vi "Run.vi"(8 "error in (no error)":errorcluster, 11 "MCCW ACLR in":refnum<class "MCCW ACLR.lvclass">) -> (0 "error out":errorcluster, 1 "Parameters":cluster{"Name":string, "Value":string}[](array[cluster]), 2 "Cancled":bool, 3 "MCCW ACLR out":refnum<class "MCCW ACLR.lvclass">)   [LabVIEW 2020, in "MCCW ACLR.lvclass"]
doc: "This is the main test vi. It is here that the test is implemented."
uses:
  MCCW ACLR.lvclass
  C:/Sandbox/RF Bench/Source Code/WiSpry Test Framework/Measurements/Measurement.lvclass
  Controls/Run States.ctl
  MCCW ACLR.lvclass/MCCW ACLR.ctl
  Instruments/Spectrum Analyzer/Spectrum Analyzer.lvclass/Spectrum Analyzer.ctl
  Measurement.lvclass/Measurement.ctl
  Devices/Controls/Change setting mode enum.ctl
  Support VI/Update parameters (single).vi
  Devices/Device.lvclass
  Instruments/Spectrum Analyzer/Spectrum Analyzer.lvclass
  Instruments/Vector Signal Generator/Vector Signal Generator.lvclass
  Measurement.lvclass
  XML Handler/XML Handler.lvclass
  Devices/PIC-device/PIC-Device.lvclass
panel:
  out "Number of Carriers":i32
  out "Device Parameters":string
  in  "Cancel Button":bool
  out "Current Frequency [Hz]":dbl format="%#_6p"
  out "Current Power [dBm]":dbl
  out "Estimated finish time":timestamp format="%<%X>T"
  out "XY Graph":cluster{dbl[], dbl[]}[](graph)
  out "Progress":u8(slide) scale=0.0..100.0
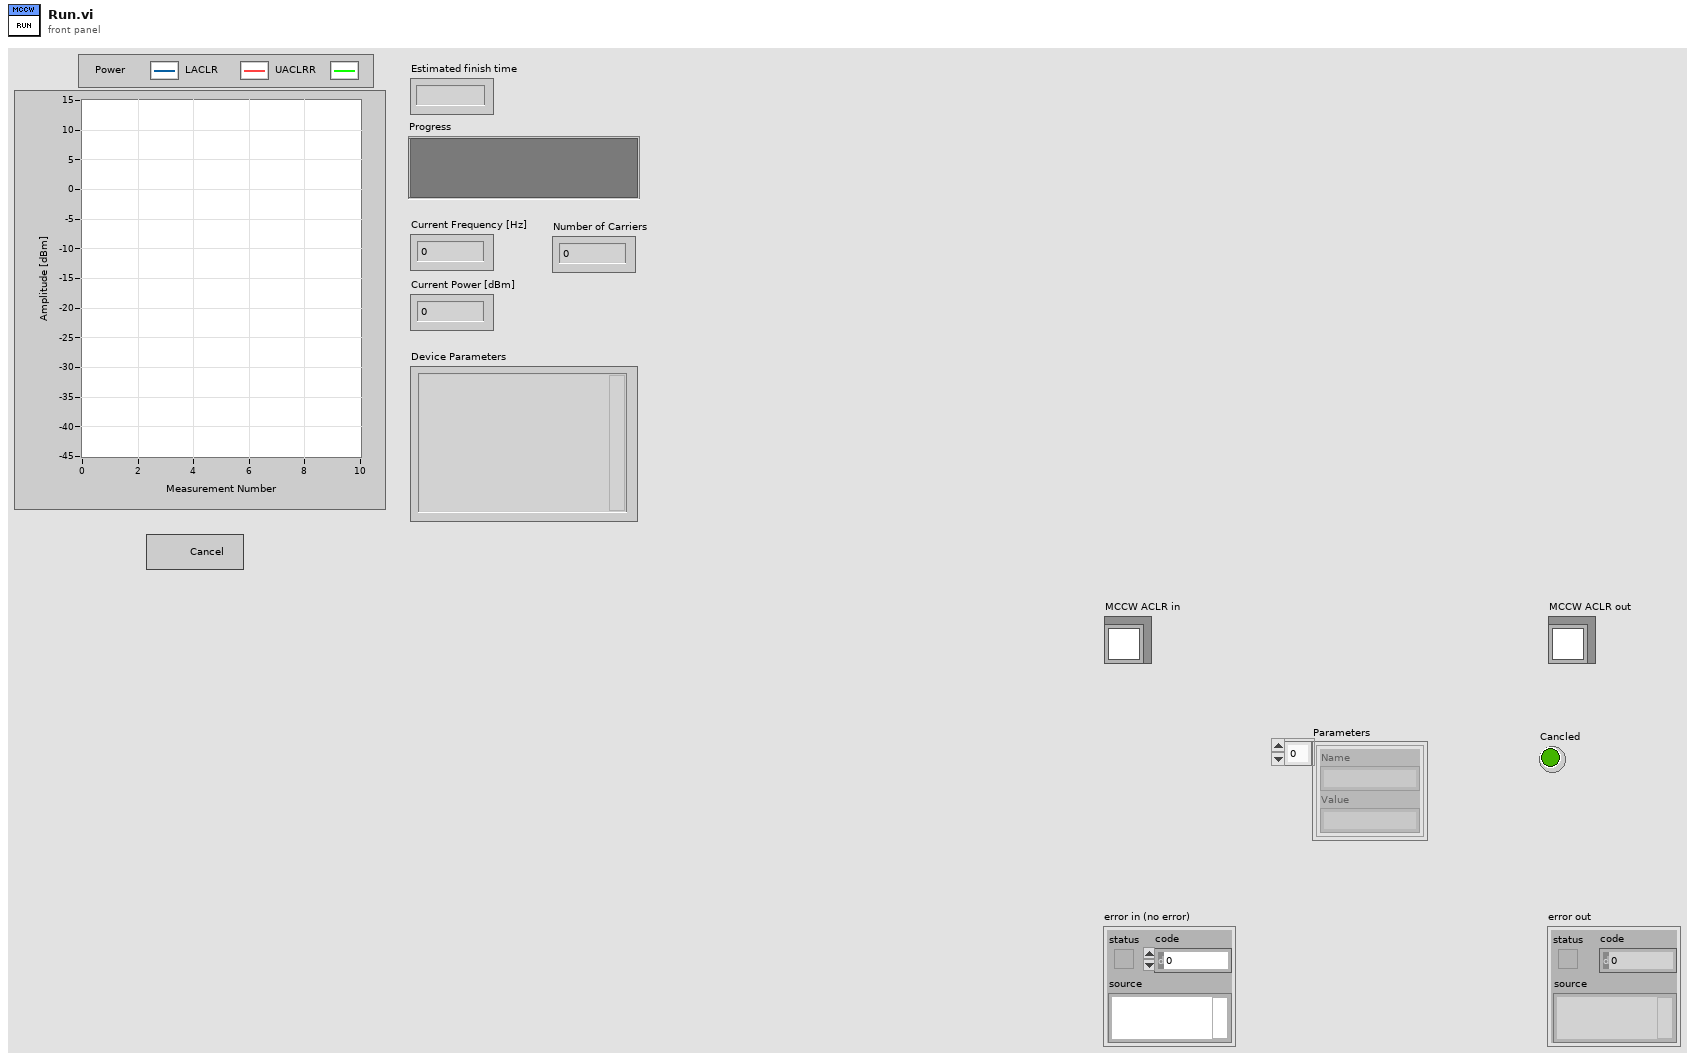
[diagram p1: front panel]
types:
  T1 = typedef "MCCW ACLR.lvclass/Run States.ctl" = enum16{"Init", "Set Frequency", "Set Power", "Set Carriers", "Set Device", "Set Measurement Number", "Measure", "Done"}
  T2 = typedef "PIC-Device.lvclass/Change setting mode enum.ctl" = enum16{"Init", "Next", "Reset"}
  T3 = typedef "MCCW ACLR.lvclass/ACLR configuration.ctl" = cluster{"Frequency":cluster{"Cluster ":cluster{"From":dbl, "To":dbl, "Step":dbl}, "Array":dbl[], "Use Array":bool}, "Power":cluster{"Cluster ":cluster{"From":dbl, "To":dbl, "Step":dbl}, "Array":dbl[], "Use Array":bool}, "Carriers":cluster{"Cluster ":cluster{"From":dbl, "To":dbl, "Step":dbl}, "Array":dbl[], "Use Array":bool}, "Phase Value":dbl, "Number of Measurements":u32, "Use random phase":bool, "Signal BW [MHz] ":dbl}
  T4 = cluster{"List":dbl[], "Index":i32, "Last":bool, "BW [MHz]":dbl}
  T5 = cluster{"Number of Measurements":u32, "Current Measurement":u32, "Last":bool}
  T6 = typedef "XML Handler.lvclass/Result Cluster.ctl" = cluster{"Name":string, "Value":string}
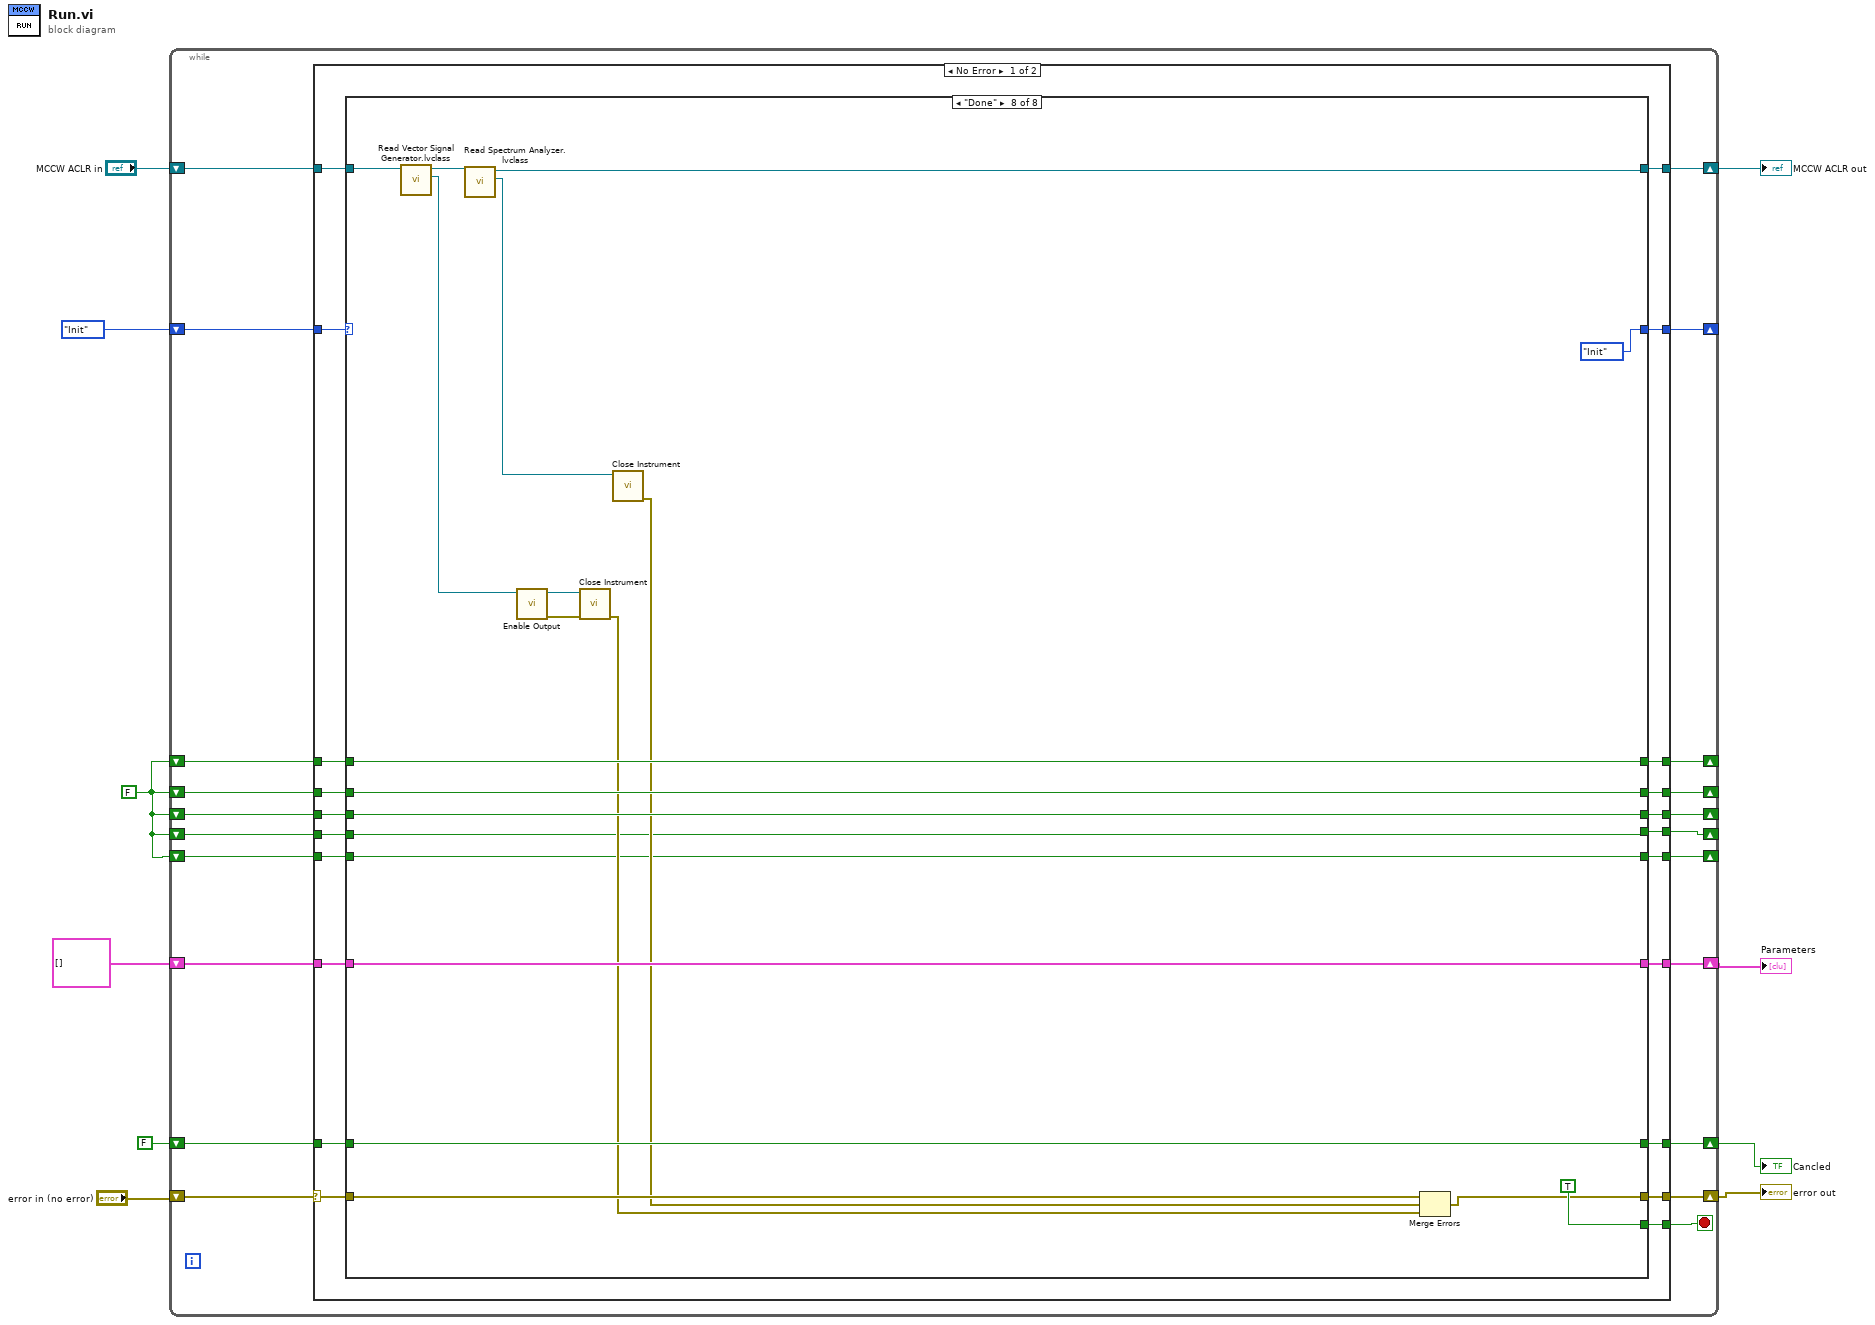
[diagram p0: block diagram]
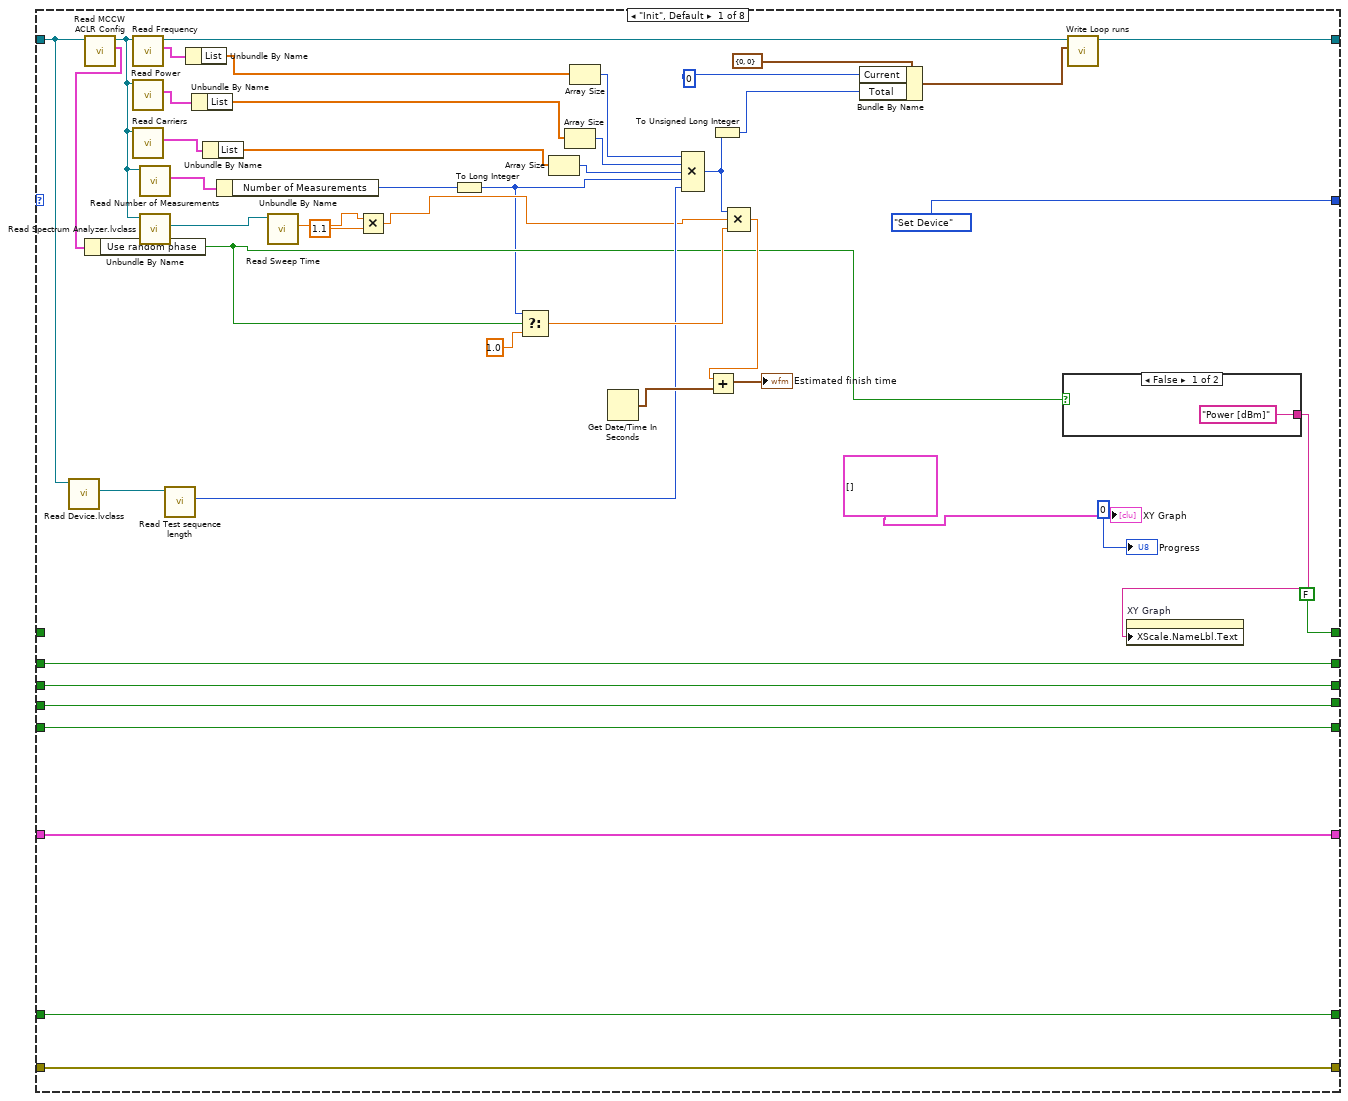
[diagram p2: hidden frame]
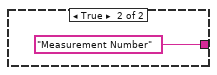
[diagram p3: hidden frame]
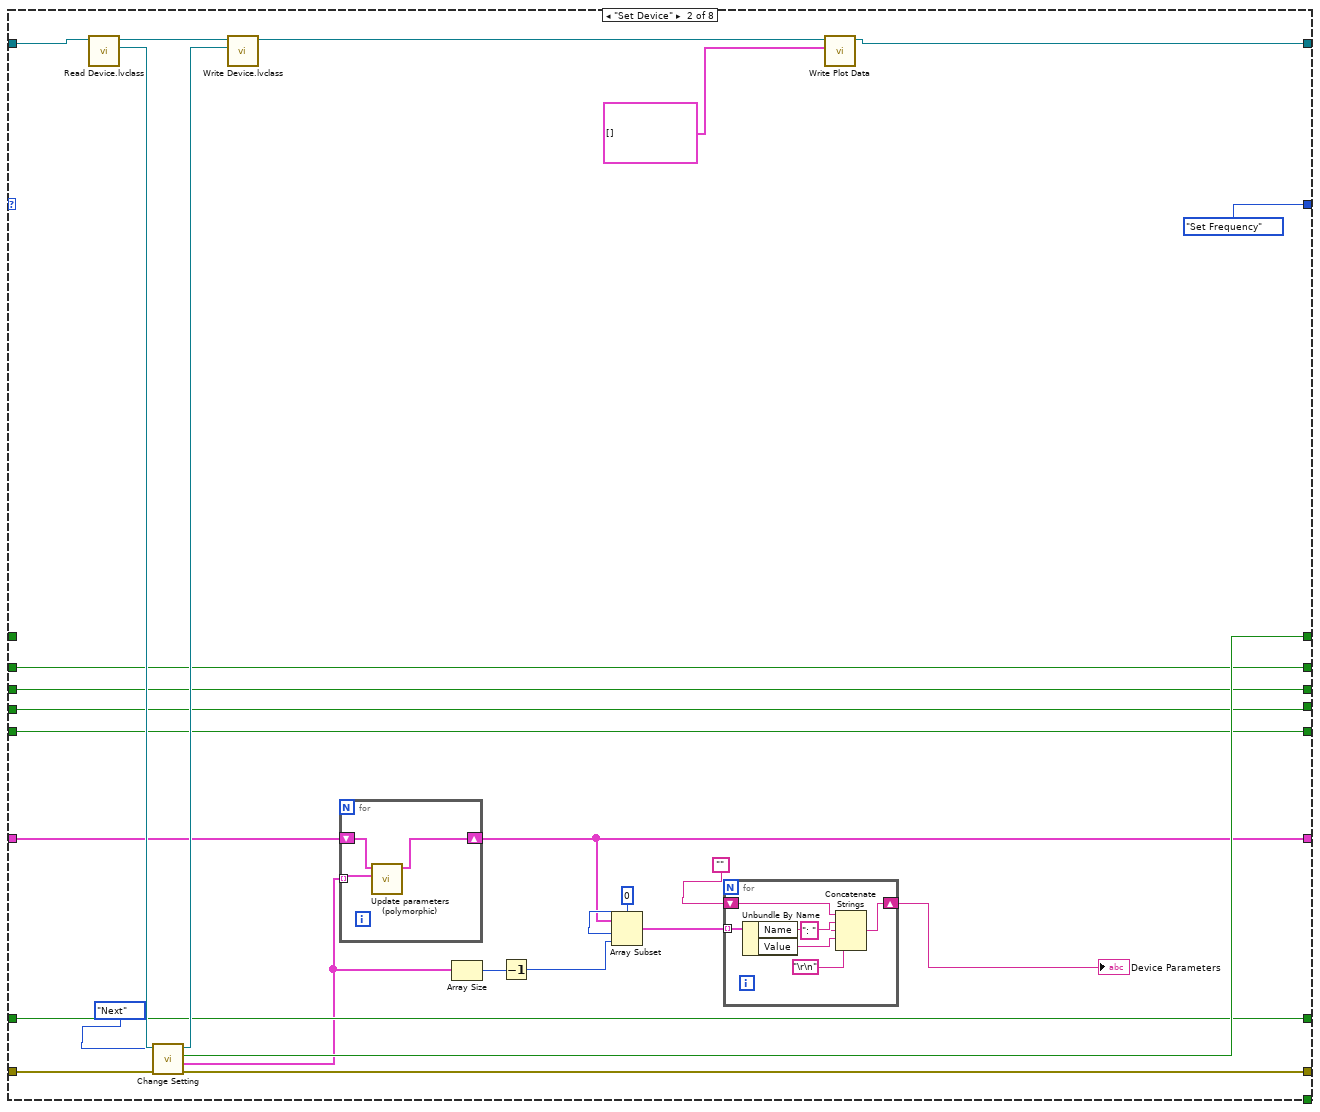
[diagram p4: hidden frame]
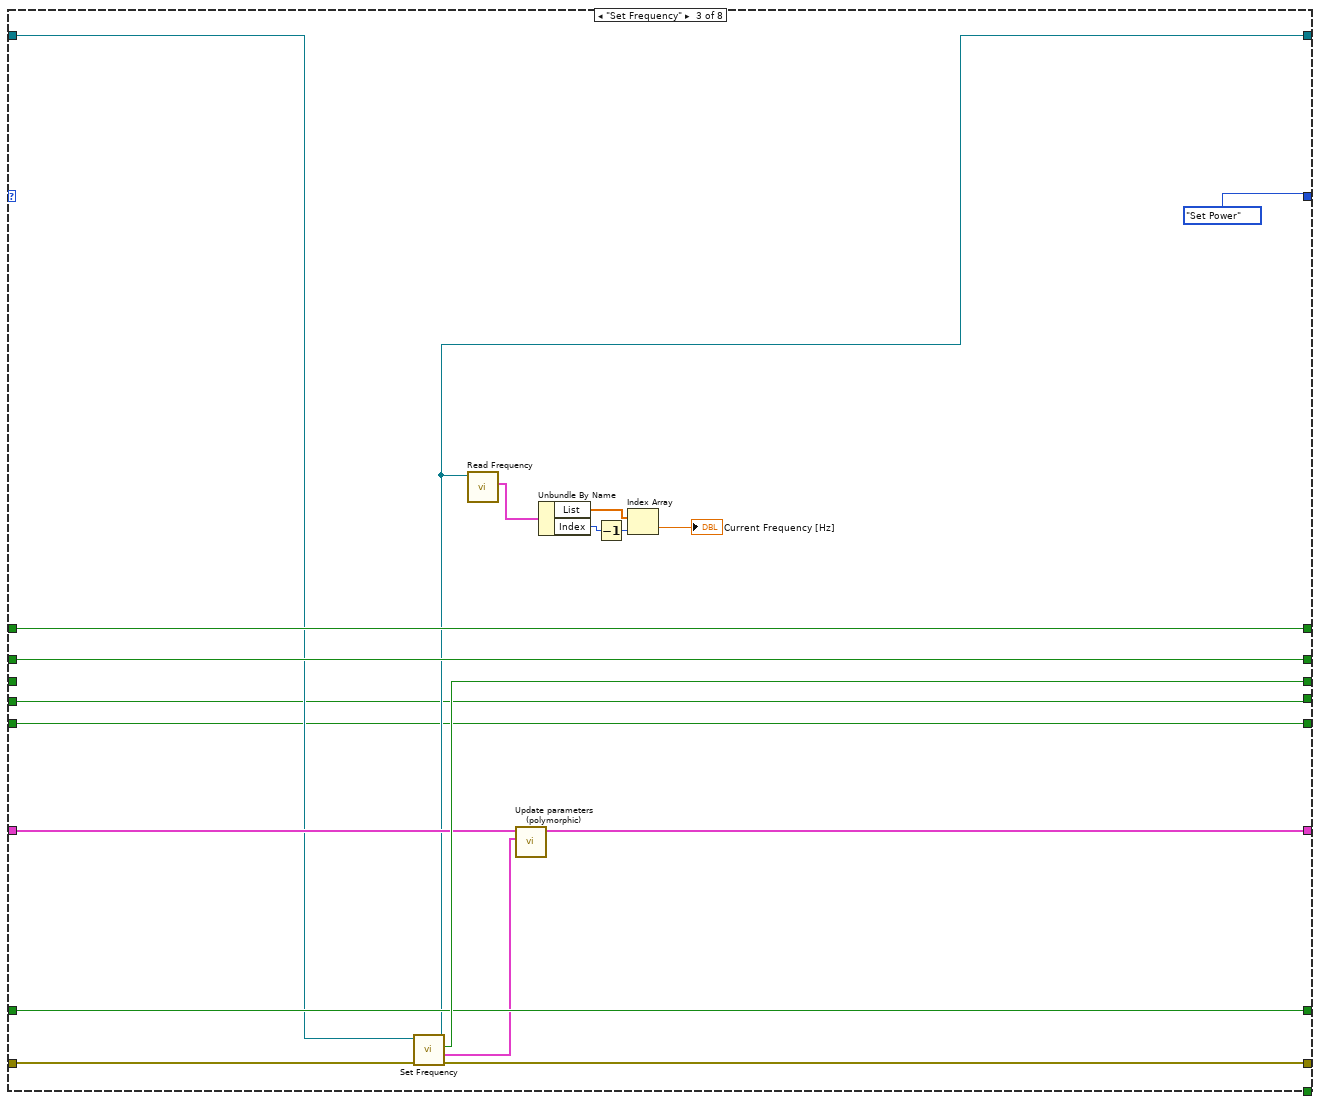
[diagram p5: hidden frame]
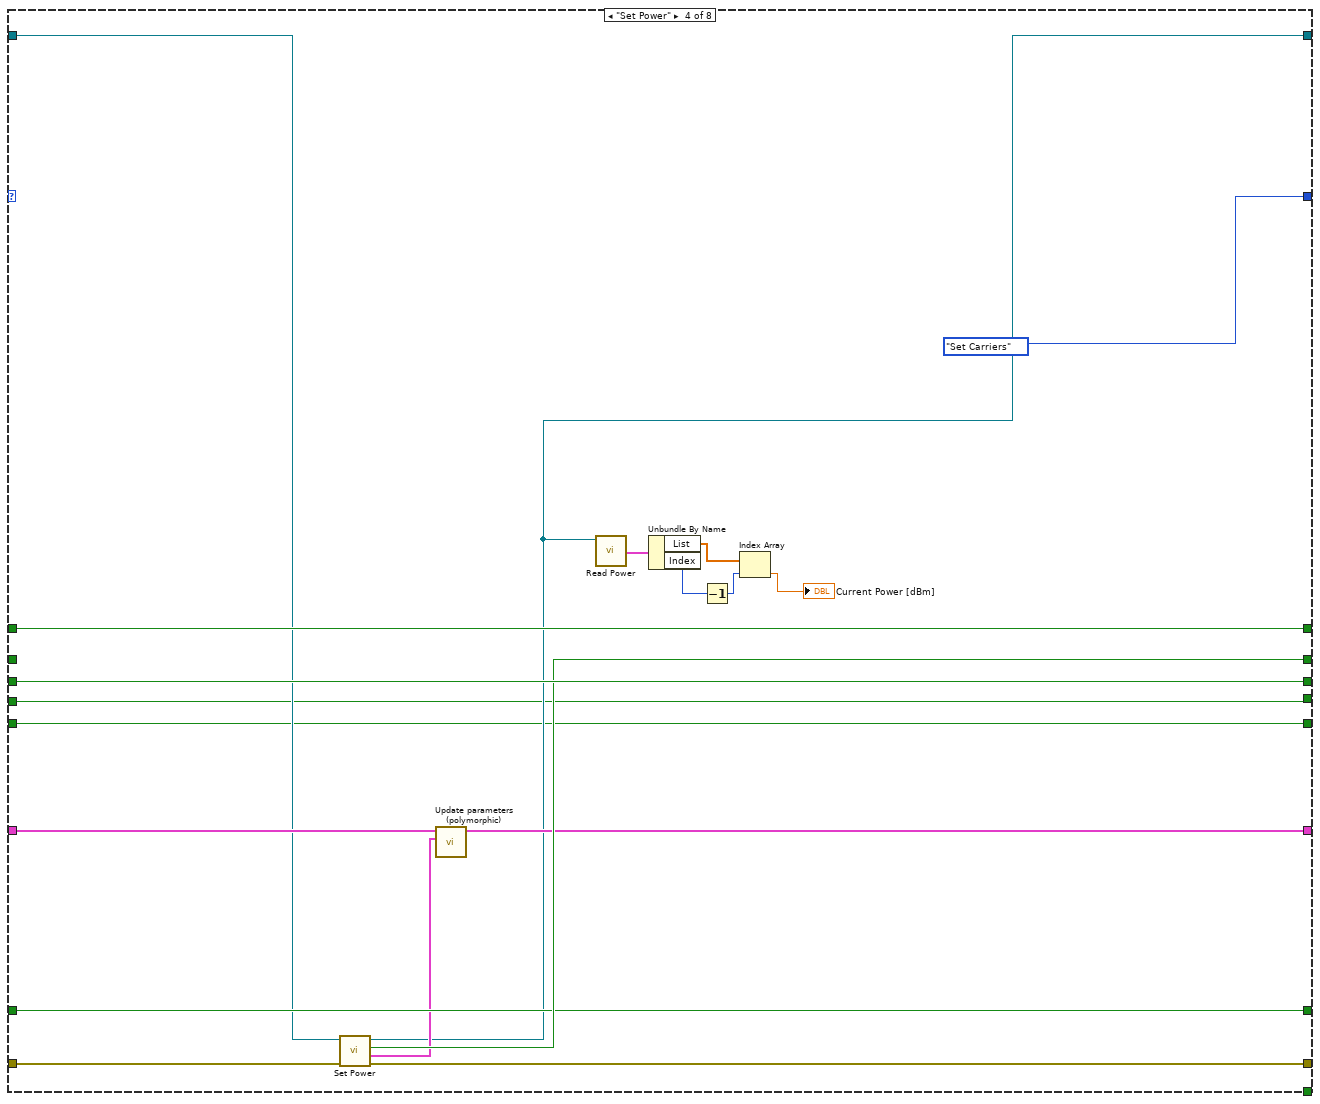
[diagram p6: hidden frame]
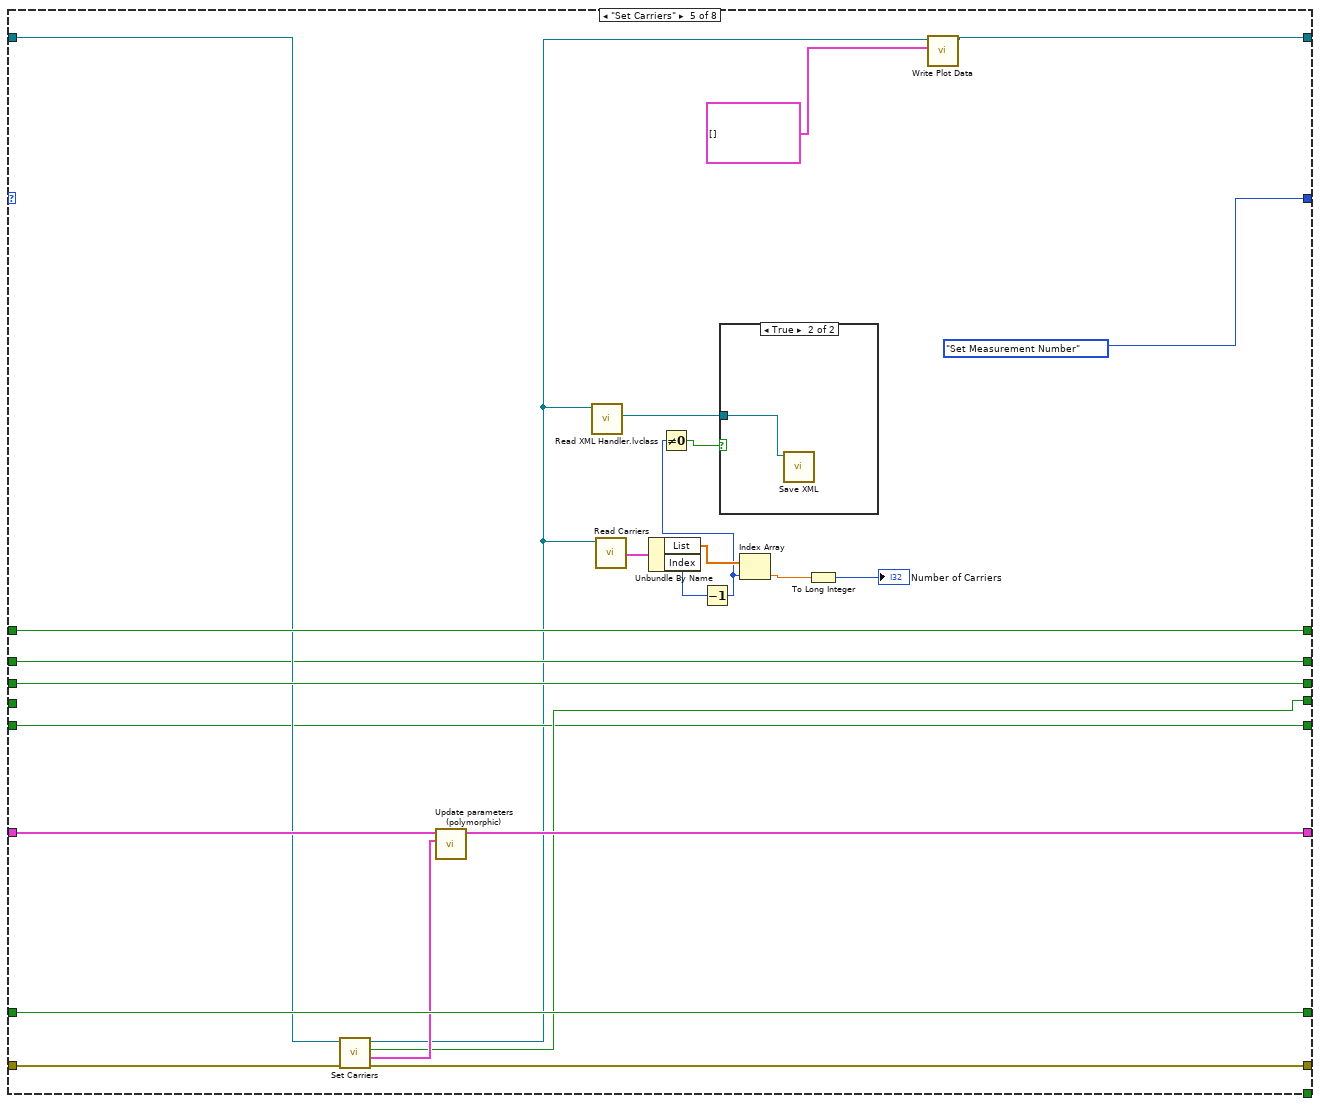
[diagram p7: hidden frame]
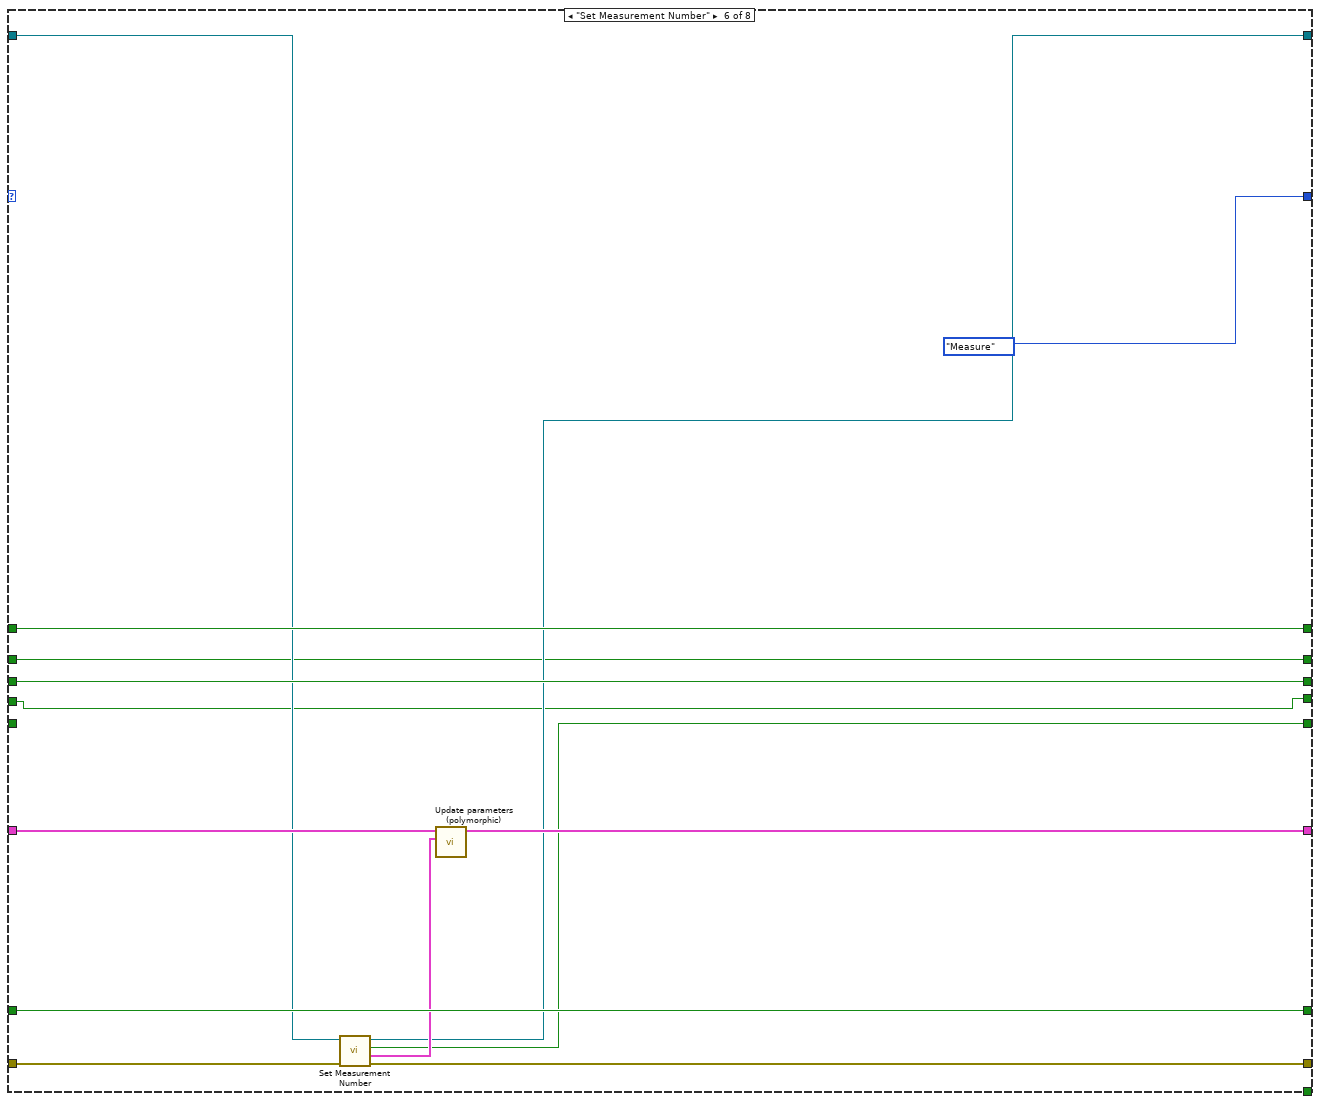
[diagram p9: hidden frame]
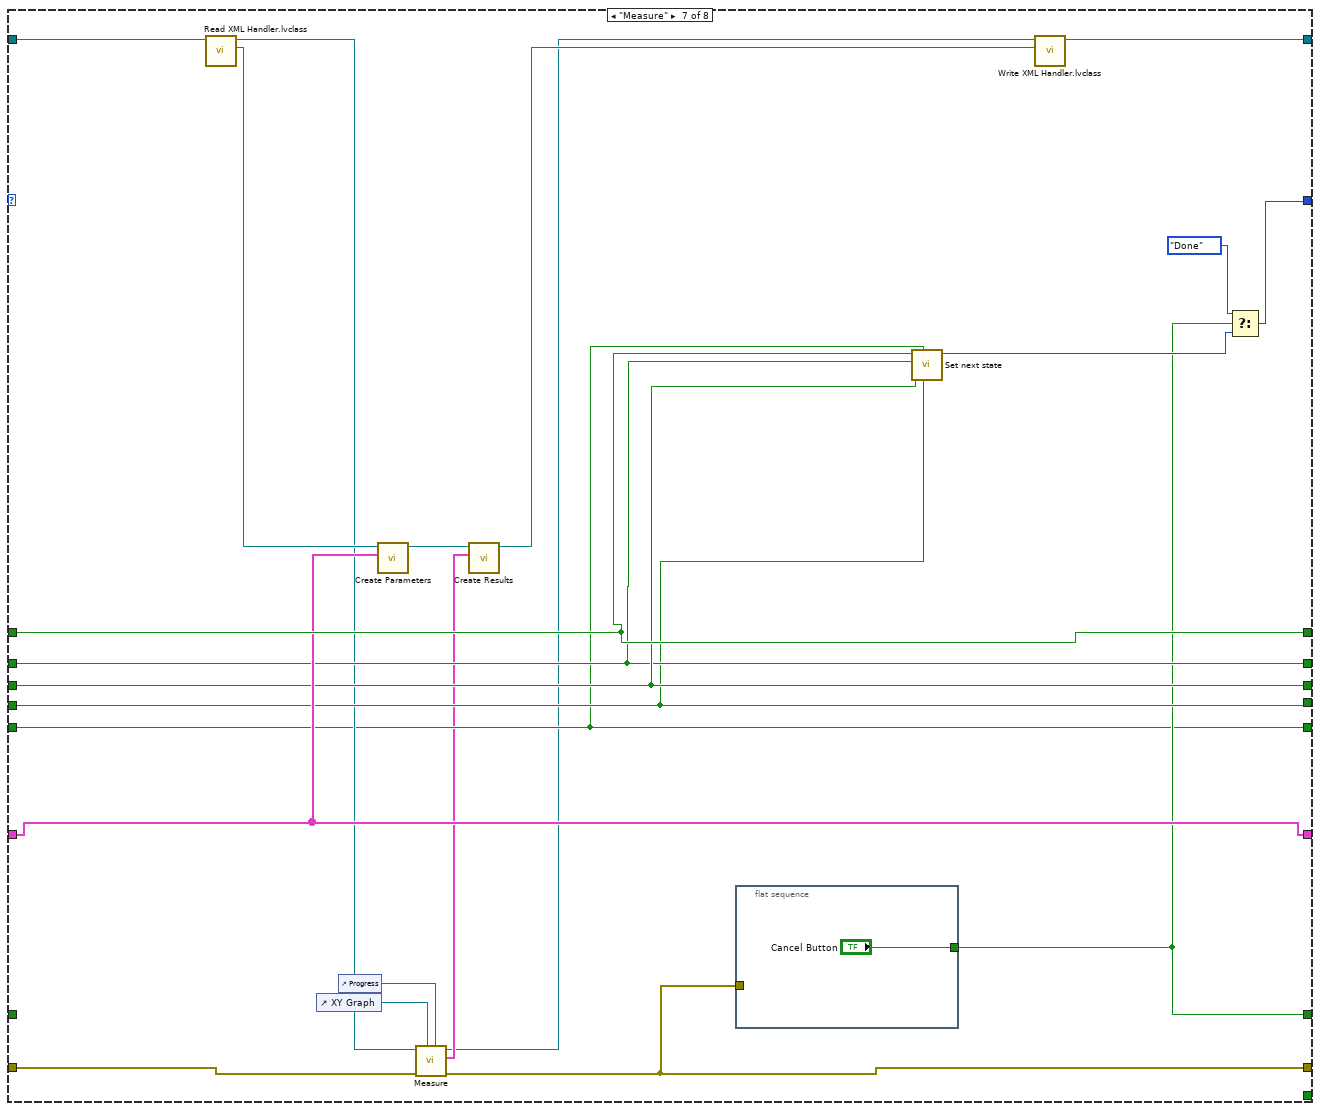
[diagram p10: hidden frame]
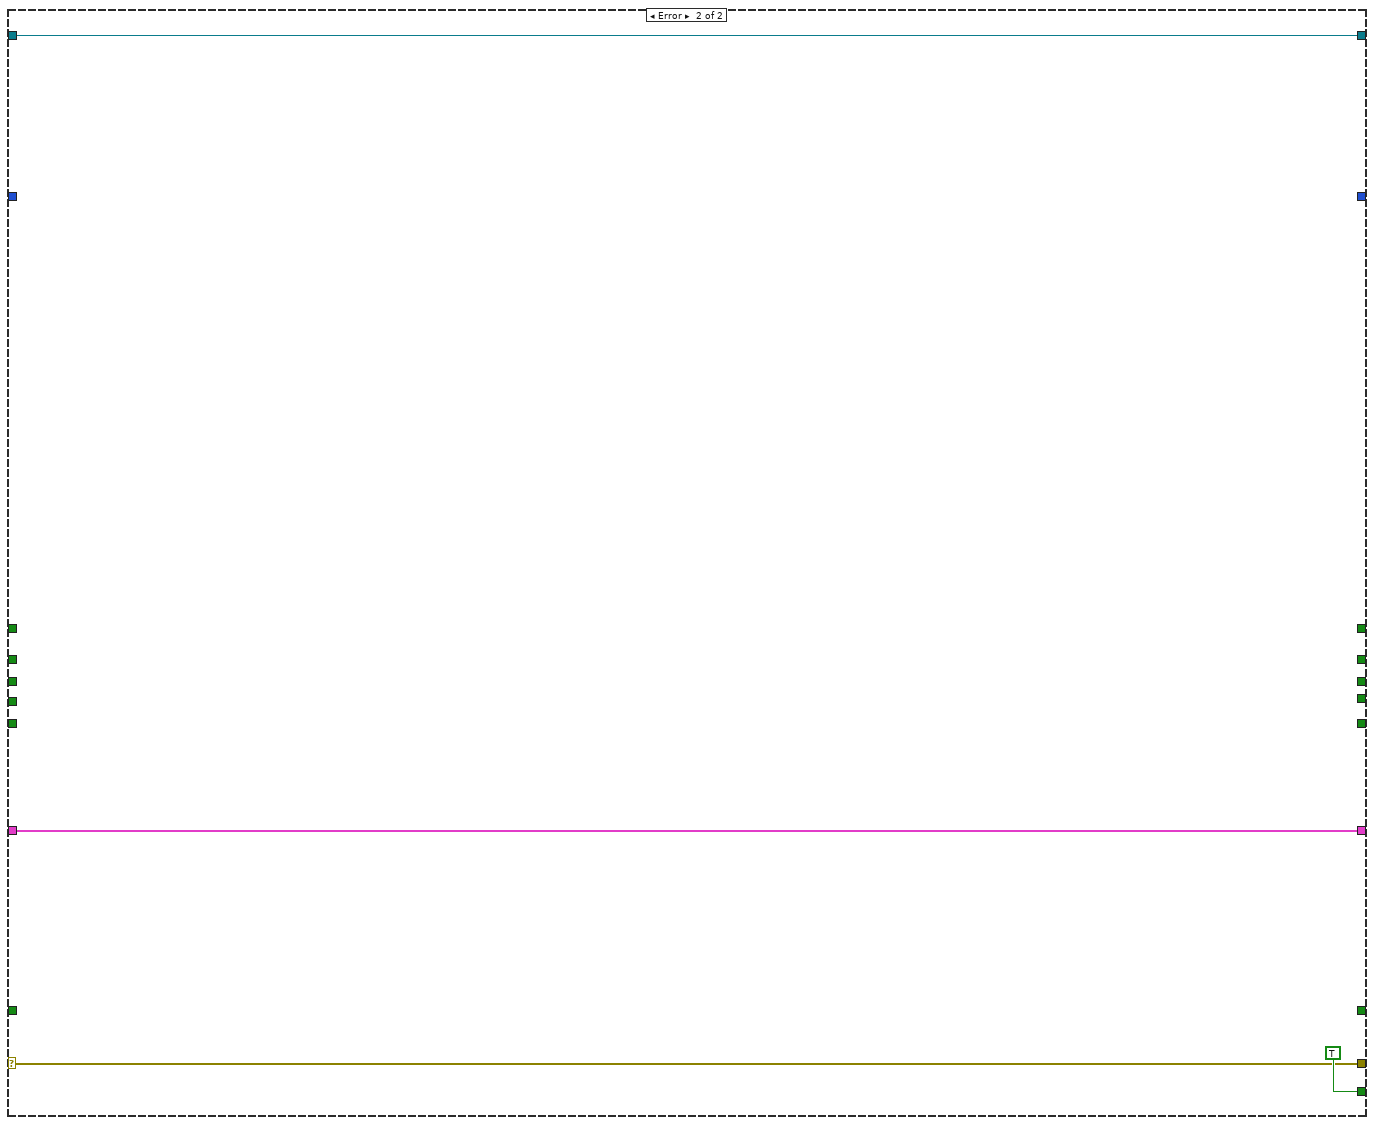
[diagram p11: hidden frame]
diagram:
  w5 = FALSE
  n1 = while {
    shift-right: [w28] -> w4
    shift-left: "error in (no error)" -> [w31]
    shift-right: [w14] -> _
    shift-left: Run_States."Init" ("Run States") -> [w30]
    shift-right: [w27] -> _
    shift-left: w5 -> [w26]
    shift-right: [w23] -> _
    shift-left: w5 -> [w25]
    shift-right: [w22] -> _
    shift-left: w5 -> [w24]
    shift-right: [w21] -> w3
    shift-left: FALSE ("Cancel Button") -> [w20]
    shift-right: [w18] -> w1
    shift-left: cluster{"Name":string, "Value":string}[] [] ("Parameters") -> [w19]
    shift-right: [w13] -> w7
    shift-left: "MCCW ACLR in" -> [w17]
    shift-right: [w15] -> _
    shift-left: w5 -> [w16]
    shift-right: [w11] -> _
    shift-left: w5 -> [w12]
    stop <- w29 stop-if-true
    n2 = case shown="No Error" w31 {
      selector: w31 -> [w50 w259]
      tunnel: w17 -> [w52 w257]
      tunnel: w30 -> [w51 _]
      tunnel: [w32 w257] -> w13
      tunnel: [w49 TRUE] -> w29
      tunnel: [w48 w259] -> w28
      tunnel: [w47 _] -> w27
      tunnel: w26 -> [w46 _]
      tunnel: [w45 _] -> w14
      tunnel: w25 -> [w44 _]
      tunnel: w24 -> [w43 _]
      tunnel: [w42 _] -> w23
      tunnel: [w41 _] -> w22
      tunnel: [w40 _] -> w21
      tunnel: w20 -> [w39 _]
      tunnel: w19 -> [w38 w258]
      tunnel: [w37 w258] -> w18
      tunnel: w16 -> [w36 _]
      tunnel: [w35 _] -> w15
      tunnel: w12 -> [w34 _]
      tunnel: [w33 _] -> w11
      frame No Error {
        n3 = case shown="\"Done\"" w51 {
          tunnel: w52 -> [w62 w126 w139 w160 w186 w205 w235 w241]
          tunnel: [w77 w103 w141 w159 w179 w204 w233 w238] -> w32
          tunnel: w50 -> [w79 w123 w153 w172 w196 w211 w222 w248]
          tunnel: [_ _ _ _ _ _ _ TRUE] -> w49
          tunnel: [w79 w116 w150 w169 w194 w209 w214 w245] -> w48
          tunnel: [FALSE ("Last setting") w121 w155 w174 w198 w213 w232 w256] -> w47
          tunnel: w46 -> [_ _ w155 w174 w198 w213 w232 w256]
          tunnel: [Run_States."Set Device" ("Run States") Run_States."Set Frequency" ("Run States") Run_States."Set Power" ("Run States") Run_States."Set Carriers" ("Run States") Run_States."Set Measurement Number" ("Run States") Run_States."Measure" ("Run States") w230 Run_States."Init" ("Run States")] -> w45
          tunnel: w44 -> [w91 w120 w154 _ w183 w202 w225 w255]
          tunnel: w43 -> [w90 w119 _ w173 w197 w212 w226 w254]
          tunnel: [w91 w120 w154 w171 w183 w202 w225 w255] -> w42
          tunnel: [w90 w119 w152 w173 w197 w212 w226 w254] -> w41
          tunnel: [w87 w118 w151 w170 w195 w210 w220 w252] -> w40
          tunnel: w39 -> [w87 w118 w151 w170 w195 w210 _ w252]
          tunnel: w38 -> [w82 w115 w149 w168 w193 w208 w227 w251]
          tunnel: [w82 w111 w148 w167 w192 w207 w227 w251] -> w37
          tunnel: w36 -> [w64 w102 w138 w157 _ w201 w224 w244]
          tunnel: [w64 w102 w138 w157 w184 w201 w224 w244] -> w35
          tunnel: w34 -> [w61 w101 w137 w156 w181 _ w217 w242]
          tunnel: [w61 w101 w137 w156 w181 w200 w217 w242] -> w33
          frame "Init", Default {
            n4 = call "Read Device.lvclass.vi"("Measurements in"=w62) -> ("Device.lvclass"=w92:refnum<class "Device.lvclass">)  [unwired: 9 in, 1 out]
            n5 = call "Read MCCW ACLR Config.vi"("MCCW ACLR in"=w62) -> ("MCCW ACLR Config"=w75:T3, "MCCW ACLR out"=w57:refnum<class "MCCW ACLR.lvclass">)  [unwired: 9 in]
            n6 = Unbundle By Name(w75) -> ("Use random phase"=w76:bool)
            n7 = call "Read Frequency.vi"("MCCW ACLR in"=w57) -> ("Frequency"=w74:cluster{"List":dbl[], "Index":i32, "Last":bool}, "MCCW ACLR out"=w63:refnum<class "MCCW ACLR.lvclass">)  [unwired: 9 in]
            n8 = call "Read Power.vi"("MCCW ACLR in"=w57) -> ("Power"=w73:cluster{"List":dbl[], "Index":i32, "Last":bool})  [unwired: 9 in, 1 out]
            n9 = call "Read Carriers.vi"("MCCW ACLR in"=w57) -> ("Carriers"=w72:T4)  [unwired: 9 in, 1 out]
            n10 = call "Read Number of Measurements.vi"("MCCW ACLR in"=w57) -> ("Number of Measurements"=w56:T5)  [unwired: 9 in, 1 out]
            n11 = call "Read Spectrum Analyzer.lvclass.vi"("MCCW ACLR in"=w57) -> ("Spectrum Analyzer.lvclass"=w67:refnum<class "Spectrum Analyzer.lvclass">)  [unwired: 9 in, 1 out]
            n12 = call-dynamic "Read Test sequence length.vi"("Device in"=w92) -> ("Test sequence length"=w93:i32)  [unwired: 8 in, 2 out]
            n13 = Unbundle By Name(w74) -> ("List"=w89:dbl[])
            n14 = Unbundle By Name(w73) -> ("List"=w88:dbl[])
            n15 = Unbundle By Name(w72) -> ("List"=w68:dbl[])
            n16 = Unbundle By Name(w56) -> ("Number of Measurements"=w55:u32)
            n17 = call "Read Sweep Time.vi"("Spectrum Analyzer in"=w67) -> ("Sweep Time"=w60:dbl)  [unwired: 9 in, 1 out]
            n18 = Multiply(x=w60, y=1.1) -> (x*y=w59:dbl)
            n19 = To Long Integer(number=w55) -> (32bit integer=w53:i32)
            n20 = Select(t=w53, s=w76, f=1.0) -> (s? t:f=w95:dbl)
            n21 = Array Size(array=w68) -> (size(s)=w69:i32)
            n22 = Array Size(array=w88) -> (size(s)=w70:i32)
            n23 = Array Size(array=w89) -> (size(s)=w71:i32)
            n24 = Get Date/Time In Seconds() -> (seconds since 1Jan1904=w98:timestamp)
            n25 = Compound Arithmetic op=MULTIPLY(w71, w70, w69, w53, w93) -> (w83:i32)
            n26 = To Unsigned Long Integer(number=w83) -> (unsigned 32bit integer=w54:u32)
            n27 = Compound Arithmetic op=MULTIPLY(w83, w59, w95) -> (w94:dbl)
            n28 = Add(x=w94, y=w98) -> (x+y=→"Estimated finish time":timestamp)
            n29 = Bundle By Name(cluster=cluster{"Current":u32, "Total":u32} {"Current"=0, "Total"=0} ("Loop runs"), "Current"=u32 0, "Total"=w54) -> (w84:cluster{"Current":u32, "Total":u32})
            n30 = case shown="False" w76 {
              tunnel: ["Power [dBm]" "Measurement Number"] -> w80
              frame False {
              }
              frame True {
              }
            }
            n31 = call "Write Loop runs.vi"("Loop runs"=w84, "Measurements in"=w63) -> ("Measurements out"=w77:refnum<class "MCCW ACLR.lvclass">)  [unwired: 9 in]
            n32 = property on="XY Graph" class="XYGraph (strict)"("XScale.NameLbl.Text"=w80) -> ()  [unwired: 2 in, 2 out]
            "XY Graph" <- cluster{dbl[], dbl[]}[] [] ("XY Graph")
            "Progress" <- u8 0 ("Progress")
          }
          frame "Set Device" {
            n33 = call "Read Device.lvclass.vi"("Measurements in"=w126) -> ("Device.lvclass"=w125:refnum<class "Device.lvclass">, "Measurements out"=w117:refnum<class "MCCW ACLR.lvclass">)  [unwired: 9 in]
            n34 = call-dynamic "Change Setting.vi"("error in (no error)"=w123, "Change setting mode"=Change_setting_mode_enum."Next", "Device in"=w125) -> ("error out"=w116:errorcluster, "Changes"=w114:cluster{"Name":string, "Value":string}[], "Last setting"=w121:bool, "Device out"=w122:refnum<class "Device.lvclass">)  [unwired: 5 in]
            n35 = call "Write Device.lvclass.vi"("Device.lvclass"=w122, "Measurements in"=w117) -> ("Measurements out"=w105:refnum<class "MCCW ACLR.lvclass">)  [unwired: 9 in]
            n36 = for {
              shift-right: [w135] -> w111
              shift-left: w115 -> [w136]
              tunnel: w114 -> [w134] mode=indexing
              n37 = call-poly "Update parameters (polymorphic).vi"("New Parameter"=w134, "Parameters"=w136) -> ("Parameters Out"=w135:cluster{"Name":string, "Value":string}[])  [unwired: 9 in]
            }
            n38 = Array Size(array=w114) -> (size(s)=w112:i32)
            n39 = Decrement(x=w112) -> (x-1=w107:i32)
            n40 = Array Subset(array=w111, index=0, length=w107) -> (w110:cluster{"Name":string, "Value":string}[])
            n41 = for {
              tunnel: w110 -> [w133] mode=indexing
              shift-right: [w127] -> w108
              shift-left: "" -> [w132]
              n42 = Unbundle By Name(w133) -> ("Name"=w131:string, "Value"=w129:string)
              n43 = Concatenate Strings(w132, w131, ": " ("string"), w129, "\r\n") -> (w127:string)
            }
            "Device Parameters" <- w108
            n44 = call "Write Plot Data.vi"("Plot Data"=cluster{"Array":dbl[], "Array":dbl[]}[] [] ("Graph Data"), "MCCW ACLR in"=w105) -> ("MCCW ACLR out"=w103:refnum<class "MCCW ACLR.lvclass">)  [unwired: 9 in]
          }
          frame "Set Frequency" {
            n45 = call "Set Frequency.vi"("error in (no error)"=w153, "MCCW ACLR in"=w139) -> ("error out"=w150:errorcluster, "Parameter"=w147:cluster{"Name":string, "Value":string}, "Last Frequency?"=w152:bool, "MCCW ACLR out"=w141:refnum<class "MCCW ACLR.lvclass">)  [unwired: 6 in]
            n46 = call "Read Frequency.vi"("MCCW ACLR in"=w141) -> ("Frequency"=w146:cluster{"List":dbl[], "Index":i32, "Last":bool})  [unwired: 9 in, 1 out]
            n47 = call-poly "Update parameters (polymorphic).vi"("New Parameter"=w147, "Parameters"=w149) -> ("Parameters Out"=w148:cluster{"Name":string, "Value":string}[])  [unwired: 9 in]
            n48 = Unbundle By Name(w146) -> ("List"=w145:dbl[], "Index"=w144:i32)
            n49 = Decrement(x=w144) -> (x-1=w143:i32)
            n50 = Index Array(array=w145, index=w143) -> (element=→"Current Frequency [Hz]":dbl)
          }
          frame "Set Power" {
            n51 = call "Set Power.vi"("error in (no error)"=w172, "MCCW ACLR in"=w160) -> ("error out"=w169:errorcluster, "Parameter"=w166:cluster{"Name":string, "Value":string}, "Last Power?"=w171:bool, "MCCW ACLR out"=w159:refnum<class "MCCW ACLR.lvclass">)  [unwired: 6 in]
            n52 = call-poly "Update parameters (polymorphic).vi"("New Parameter"=w166, "Parameters"=w168) -> ("Parameters Out"=w167:cluster{"Name":string, "Value":string}[])  [unwired: 9 in]
            n53 = call "Read Power.vi"("MCCW ACLR in"=w159) -> ("Power"=w165:cluster{"List":dbl[], "Index":i32, "Last":bool})  [unwired: 9 in, 1 out]
            n54 = Unbundle By Name(w165) -> ("List"=w163:dbl[], "Index"=w161:i32)
            n55 = Decrement(x=w161) -> (x-1=w162:i32)
            n56 = Index Array(array=w163, index=w162) -> (element=→"Current Power [dBm]":dbl)
          }
          frame "Set Carriers" {
            n57 = call "Set Carriers.vi"("error in (no error)"=w196, "MCCW ACLR in"=w186) -> ("error out"=w194:errorcluster, "Parameter"=w191:cluster{"Name":string, "Value":string}, "Last Carrier?"=w184:bool, "MCCW ACLR out"=w176:refnum<class "MCCW ACLR.lvclass">)  [unwired: 6 in]
            n58 = call-poly "Update parameters (polymorphic).vi"("New Parameter"=w191, "Parameters"=w193) -> ("Parameters Out"=w192:cluster{"Name":string, "Value":string}[])  [unwired: 9 in]
            n59 = call "Read XML Handler.lvclass.vi"("Measurements in"=w176) -> ("XML Handler.lvclass"=w175:refnum<class "XML Handler.lvclass">)  [unwired: 9 in, 1 out]
            n60 = call "Read Carriers.vi"("MCCW ACLR in"=w176) -> ("Carriers"=w190:T4)  [unwired: 9 in, 1 out]
            n61 = Unbundle By Name(w190) -> ("List"=w188:dbl[], "Index"=w187:i32)
            n62 = Decrement(x=w187) -> (x-1=w178:i32)
            n63 = Not Equal To 0?(x=w178) -> (x != 0?=w177:bool)
            n64 = case shown="True" w177 {
              tunnel: w175 -> [_ w199]
              frame False {
              }
              frame True {
                n65 = call "Save XML.vi"("XML Handler in"=w199) -> ()  [unwired: 9 in, 2 out]
              }
            }
            n66 = Index Array(array=w188, index=w178) -> (element=w189:dbl)
            n67 = To Long Integer(number=w189) -> (32bit integer=→"Number of Carriers":i32)
            n68 = call "Write Plot Data.vi"("Plot Data"=cluster{"Array":dbl[], "Array":dbl[]}[] [] ("Graph Data"), "MCCW ACLR in"=w176) -> ("MCCW ACLR out"=w179:refnum<class "MCCW ACLR.lvclass">)  [unwired: 9 in]
          }
          frame "Set Measurement Number" {
            n69 = call "Set Measurement Number.vi"("error in (no error)"=w211, "MCCW ACLR in"=w205) -> ("error out"=w209:errorcluster, "Parameter"=w206:cluster{"Name":string, "Value":string}, "Last Carrier?"=w200:bool, "MCCW ACLR out"=w204:refnum<class "MCCW ACLR.lvclass">)  [unwired: 6 in]
            n70 = call-poly "Update parameters (polymorphic).vi"("New Parameter"=w206, "Parameters"=w208) -> ("Parameters Out"=w207:cluster{"Name":string, "Value":string}[])  [unwired: 9 in]
          }
          frame "Measure" {
            n71 = call "Read XML Handler.lvclass.vi"("Measurements in"=w235) -> ("XML Handler.lvclass"=w229:refnum<class "XML Handler.lvclass">, "Measurements out"=w221:refnum<class "MCCW ACLR.lvclass">)  [unwired: 9 in]
            n72 = control-ref of="XY Graph"() -> (w218:refnum<vi>)
            n73 = control-ref of="Progress"() -> (w219:refnum<vi>)
            n74 = call "Create Parameters.vi"("Parameters"=w227, "XML Handler in"=w229) -> ("XML Handler out"=w228:refnum<class "XML Handler.lvclass">)  [unwired: 8 in, 1 out]
            n75 = call "Measure.vi"("Progress Ref"=w219, "XY Graph Reference"=w218, "error in (no error)"=w222, "MCCW ACLR in"=w221) -> ("error out"=w214:errorcluster, "Results"=w216:T6[], "MCCW ACLR out"=w215:refnum<class "MCCW ACLR.lvclass">)  [unwired: 5 in]
            n76 = call "Create Results.vi"("Results"=w216, "XML Handler in"=w228) -> ("XML Handler out"=w234:refnum<class "XML Handler.lvclass">)  [unwired: 8 in, 1 out]
            n77 = flat-sequence {
              tunnel: ["Cancel Button"] -> w220
              tunnel: w214 -> [_]
              frame #0 {
              }
            }
            n78 = call "Set next state.vi"("Last Carrier?"=w224, "Last Measurement"=w217, "Last Frequency?"=w226, "Last Power?"=w225, "Last setting"=w232) -> ("Run States"=w231:T1)  [unwired: 6 in]
            n79 = call "Write XML Handler.lvclass.vi"("XML Handler.lvclass"=w234, "Measurements in"=w215) -> ("Measurements out"=w233:refnum<class "MCCW ACLR.lvclass">)  [unwired: 9 in]
            n80 = Select(t=Run_States."Done" ("Run States"), s=w220, f=w231) -> (s? t:f=w230:T1)
          }
          frame "Done" {
            n81 = call "Read Vector Signal Generator.lvclass.vi"("MCCW ACLR in"=w241) -> ("Vector Signal Generator.lvclass"=w240:refnum<class "Vector Signal Generator.lvclass">, "MCCW ACLR out"=w239:refnum<class "MCCW ACLR.lvclass">)  [unwired: 9 in]
            n82 = call "Read Spectrum Analyzer.lvclass.vi"("MCCW ACLR in"=w239) -> ("Spectrum Analyzer.lvclass"=w237:refnum<class "Spectrum Analyzer.lvclass">, "MCCW ACLR out"=w238:refnum<class "MCCW ACLR.lvclass">)  [unwired: 9 in]
            n83 = call-dynamic "Enable Output.vi"("Signal Generator in"=w240) -> ("error out"=w249:errorcluster, "Signal Generator out"=w250:refnum<class "Vector Signal Generator.lvclass">)  [unwired: 9 in]
            n84 = call-dynamic "Close Instrument.vi"("error in (no error)"=w249, "Instrument in"=w250) -> ("error out"=w246:errorcluster)  [unwired: 8 in, 1 out]
            n85 = call-dynamic "Close Instrument.vi"("Instrument in"=w237) -> ("error out"=w247:errorcluster)  [unwired: 9 in, 1 out]
            n86 = Merge Errors(w248, w247, w246) -> (w245:errorcluster)
          }
        }
      }
      frame Error {
      }
    }
  }
  "error out" <- w4
  "MCCW ACLR out" <- w7
  "Cancled" <- w3
  "Parameters" <- w1
